vi "BenchConfig_Read.vi"(8 "error in (no error)":errorcluster) -> (0 "error out":errorcluster, 3 "BenchConfig":T1)   [LabVIEW 2013]
uses:
  BenchConfig.ctl
panel:
  # "A configurer"
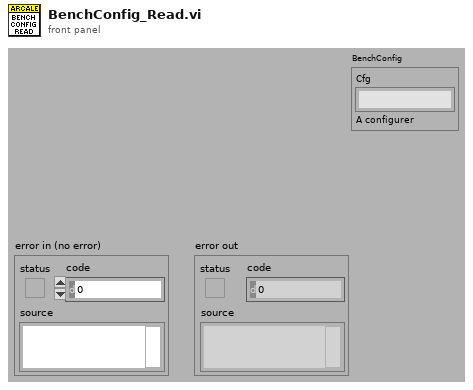
[diagram p1: front panel]
types:
  T1 = typedef "BenchConfig.ctl" = cluster{"Cfg":string}
  T2 = enum16{"open", "replace", "create", "open or create", "replace or create", "replace or create with confirmation"}
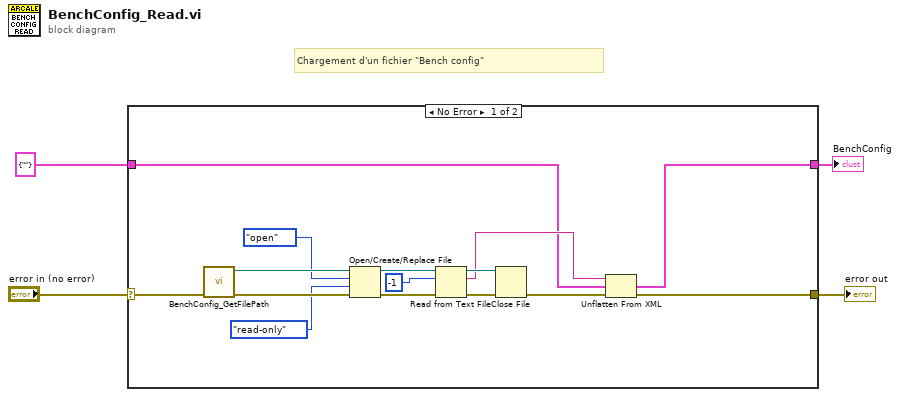
[diagram p0: block diagram]
diagram:
  # "Chargement d'un fichier \"Bench config\""
  n1 = case shown="No Error" "error in (no error)" {
    selector: "error in (no error)" -> [w19 w21]
    tunnel: [w6 w21] -> w3
    tunnel: T1 {"Cfg"=""} ("BenchConfig") -> [w7 w20]
    tunnel: [w5 w20] -> w1
    frame No Error {
      n2 = call "BenchConfig_GetFilePath.vi"("error in (no error)"=w19) -> ("error out"=w18:errorcluster, "BenchConfigFilePath"=w17:path)  [unwired: 9 in]
      n3 = Open/Create/Replace File(file path (use dialog)=w17, error in=w18, operation (0:open)=T2."open", access (0:read/write)=enum16{"read/write", "read-only", "write-only"}."read-only") -> (refnum out=w13:refnum<file>, error out=w14:errorcluster)  [unwired: 2 in, 1 out]
      n4 = Read from Text File(file (use dialog)=w13, count=-1, error in=w14) -> (refnum out=w11:refnum<file>, text=w9:string, error out=w12:errorcluster)  [unwired: 1 in, 1 out]
      n5 = Close File(refnum=w11, error in=w12) -> (error out=w8:errorcluster)  [unwired: 1 out]
      n6 = Unflatten From XML(xml string=w9, type=w7, error in (no error)=w8) -> (value=w5:T1, error out=w6:errorcluster)
    }
    frame Error {
    }
  }
  "error out" <- w3
  "BenchConfig" <- w1
